vi "PH_Synchrolock_Watch.check Limits.vi"(0 "i ref in":refnum<vi>, 5 "error in":errorcluster) -> (12 "Phase above Limit?":bool, 13 "MIRA above Limit?":bool, 14 "i ref out":refnum<vi>, 15 "Phase in range?":bool, 16 "RF Amplitude below Limit?":bool, 17 "MIRA Amplitude in range?":bool, 19 "error out":errorcluster)   [LabVIEW 2014, in "PH_Synchrolock_Watch.lvlib"]
doc: "This VI calculates whether the different values are in range ..."
uses:
  PH_Synchrolock_Watch.lvlib
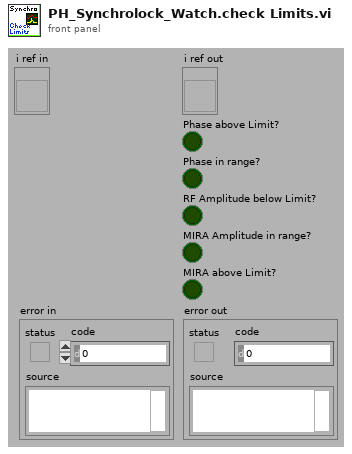
[diagram p1: front panel]
types:
  T1 = typedef "PH_Synchrolock_Watch.lvlib/PH_Synchrolock_Watch.i attribute.ctl" = cluster{"GUI Refs":cluster{"Mean Phase Graph":refnum<vi>, "RF Amplitude Graph":refnum<vi>, "Mira Amplitude Graph":refnum<vi>, "MIRA State":refnum<vi>, "Mean Phase":refnum<vi>, "RF Amplitude":refnum<vi>, "Mira Amplitude":refnum<vi>, "Mean Phase in range?":refnum<vi>, "RF Amplitude above limit?":refnum<vi>, "Mira Amplitude in range?":refnum<vi>, "Mean phase upper limit":refnum<vi>, "Mean phase lower limit":refnum<vi>, "RF Amplitude lower limit":refnum<vi>, "Mira Amplitude lower limit":refnum<vi>, "Mira Amplitude upper limit":refnum<vi>, "Waveform End":refnum<vi>, "Mira scope":refnum<vi>, "Reset Mira warning":refnum<vi>}, "Status":cluster{"Reset Warning":bool}, "Mean Phase":cluster{"Current Value":dbl, "Upper Limit":dbl, "Lower Limit":dbl, "Data":cluster{dbl[], dbl[]}}, "RF":cluster{"Current Value":dbl, "Lower Limit":dbl, "Data":cluster{dbl[], dbl[]}}, "MIRA":cluster{"Current Value":dbl, "Upper Limit":dbl, "Lower Limit":dbl, "Data":cluster{dbl[], dbl[]}}, "Waveform End":i32}
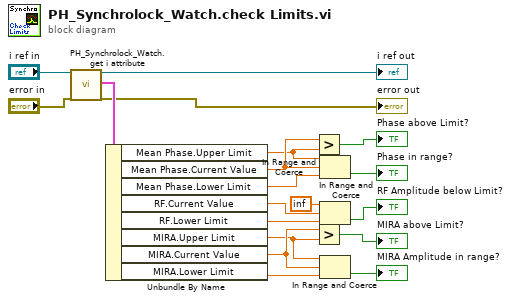
[diagram p0: block diagram]
diagram:
  n1 = call "PH_Synchrolock_Watch.get i attribute.vi"("i ref in"="i ref in", "error in (no error)"="error in") -> ("i ref out"=→"i ref out":refnum<vi>, "i attribute"=w17:T1, "error out"=→"error out":errorcluster)  [unwired: 15 in]
  n2 = Unbundle By Name(w17) -> ("Mean Phase.Upper Limit"=w5:dbl, "Mean Phase.Current Value"=w6:dbl, "Mean Phase.Lower Limit"=w16:dbl, "RF.Current Value"=w15:dbl, "RF.Lower Limit"=w13:dbl, "MIRA.Upper Limit"=w2:dbl, "MIRA.Current Value"=w3:dbl, "MIRA.Lower Limit"=w12:dbl)
  n3 = Greater?(x=w6, y=w5) -> (0:→"Phase above Limit?":bool)
  n4 = Greater?(x=w3, y=w2) -> (0:→"MIRA above Limit?":bool)
  n5 = In Range and Coerce(upper limit=w5, x=w6, lower limit=w16) -> (In Range?=→"Phase in range?":bool)  [unwired: 1 out]
  n6 = In Range and Coerce(upper limit=inf, x=w15, lower limit=w13) -> (In Range?=→"RF Amplitude below Limit?":bool)  [unwired: 1 out]
  n7 = In Range and Coerce(upper limit=w2, x=w3, lower limit=w12) -> (In Range?=→"MIRA Amplitude in range?":bool)  [unwired: 1 out]
